vi "SCM2.vi"(2 "Magnet ID":i32(ring)=16 items=["None", "Cell 12", "Cell 15", "Cell 15insert", "Cell 4", "Cell 4-2", "Cell 4-3", "Cell 5", "Cell 6", "Cell 6-2", "Cell 6-3", "Cell 7", "Cell 8", "Cell 9", "Outsert", "SCM1", "SCM2"], 4 "Keithley GPIB Address":refnum<visa-resource-name>="GPIB0::12::INSTR") -> ()   [LabVIEW 2021]
uses:
  Globals and TypeDefs/gHField.vi
  Instance           3 12Saved   SCM2 .vi
panel:
  out "Field":dbl(graph)
  in  "stop":bool
  in  "Refresh Time (s)":dbl=1.0
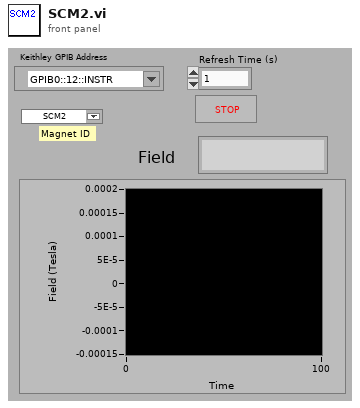
[diagram p1: front panel]
types:
  T1 = cluster{"Current Scale Factor kA/V":dbl, "I->B":dbl[], "B->I":dbl[]}
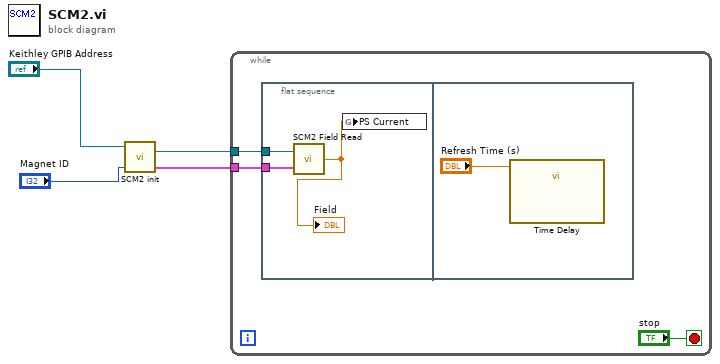
[diagram p0: block diagram]
diagram:
  n1 = call "SCM2 init.vi"("Magnet ID"="Magnet ID", "Keithley GPIB Address"="Keithley GPIB Address") -> ("Calibration"=w1:T1, "Keithley GPIB output"=w2:refnum<visa-resource-name>)  [unwired: 1 in]
  n2 = while {
    tunnel: w2 -> [w7]
    tunnel: w1 -> [w6]
    stop <- "stop" stop-if-true
    n3 = flat-sequence {
      tunnel: w7 -> [w10]
      tunnel: w6 -> [w9]
      frame #0 {
        n4 = call "SCM2 Field Read.vi"("Calibration"=w9, "Keithley GPIB Address"=w10) -> ("SCM2 Field"=w8:dbl)
        "Field" <- w8
        n5 = global write "gHField.vi" "PS Current"(w8) -> ()
      }
      frame #1 {
        n6 = call "Time Delay"("Delay Time (s)"="Refresh Time (s)") -> ()  [unwired: 10 in, 1 out]
      }
    }
  }
